vi "Reacquire Image.vi"(6 "Console Log in":refnum<class "Console Log.lvclass">, 7 "Gantry in":refnum<class "Gantry Class.lvclass">, 8 "error in":errorcluster, 10 "Chuck":i32, 11 "Fiducial Image In":T2) -> (0 "error out":errorcluster, 3 "Fiducial Image Out":T2, 4 "Console Log out":refnum<class "Console Log.lvclass">, 5 "Gantry out":refnum<class "Gantry Class.lvclass">)   [LabVIEW 2011]
uses:
  Shared Components/Utils/Type Definitions/Fiducial Image.ctl
  Shared Components/Vec3d Class/Vec3d Class.lvclass
  Shared Components/Utils/Type Definitions/Physical Image.ctl
  <vilib>/vision/Image Controls.llb/IMAQ Image.ctl
  Shared Components/Utils/Type Definitions/Fiducial with Source.ctl
  Shared Components/Gantry Class/Gantry Class.lvclass
  UI Classes/Console Log/Console Log.lvclass
  Shared Components/Config Manager Class/Type Definitions/Camera Enum.ctl
panel:
  out "Current Position":cluster{"X":dbl, "Y":dbl, "Z":dbl}
  in  "Accept":bool
  out "Preview":T1(plugin-control)
  # "Use MPG To locate fiducial\nand bring it into focus.\n\nClick \"Accept\" when\nsatisfied."
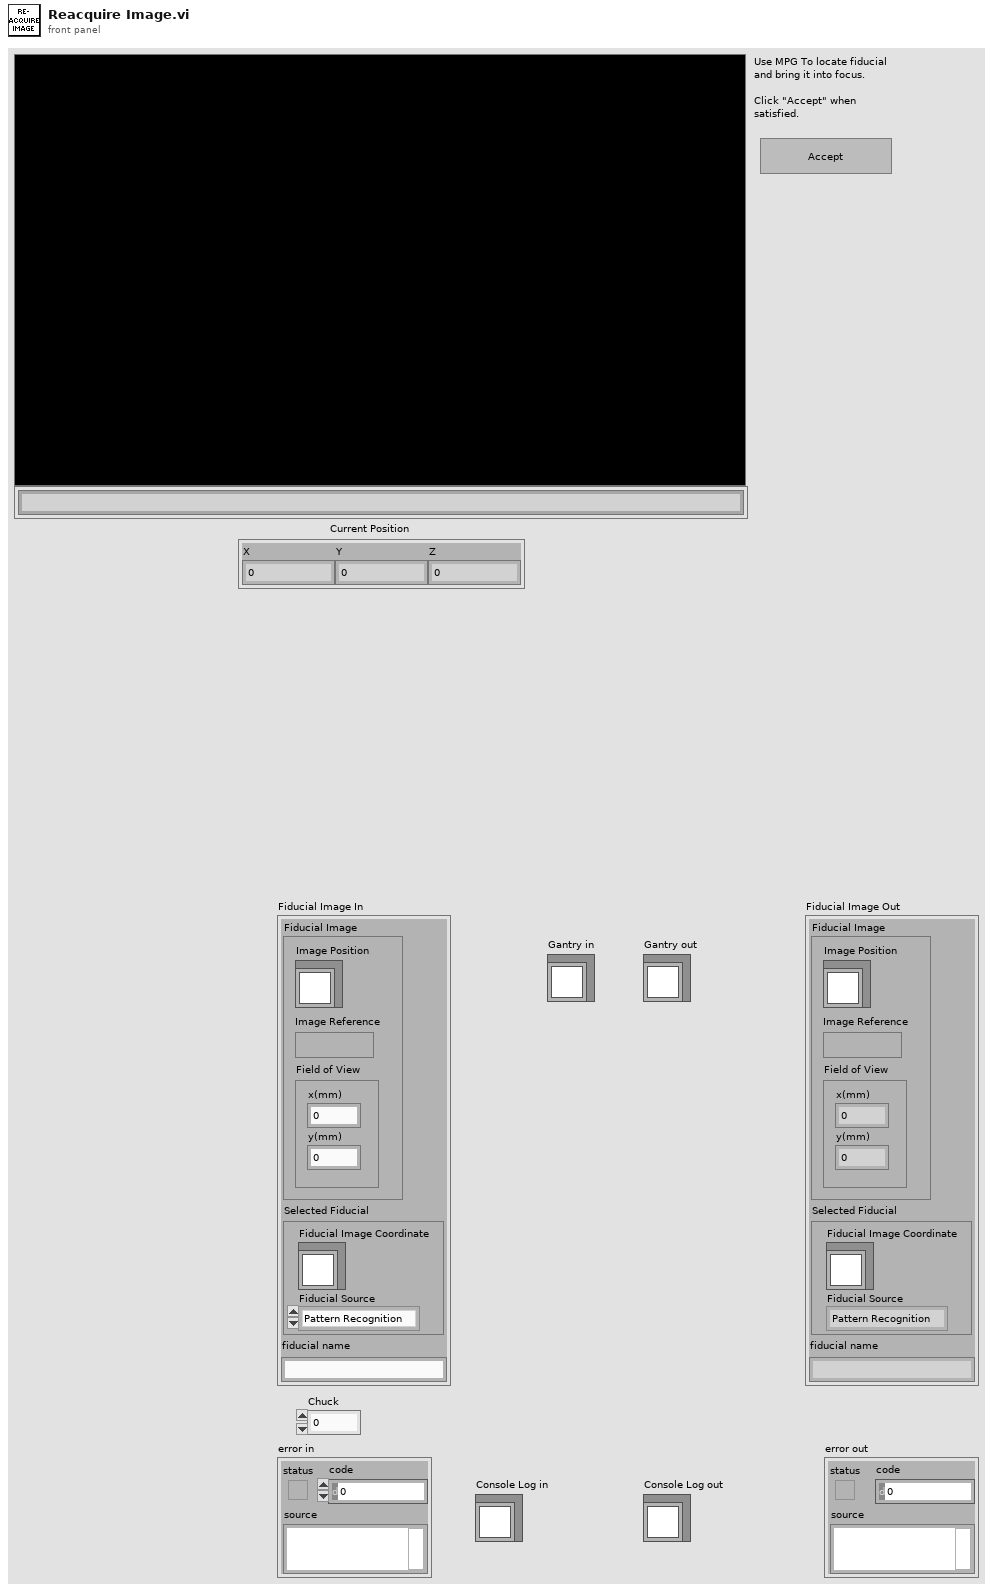
[diagram p1: front panel]
types:
  T1 = typedef "IMAQ Image.ctl" = refnum<image>
  T2 = typedef "Fiducial Image.ctl" = cluster{"Fiducial Image":T3, "Selected Fiducial":T4, "fiducial name":string}
  T3 = typedef "Physical Image.ctl" = cluster{"Image Position":refnum<class "Vec3d Class.lvclass">, "Image Reference":T1, "Field of View":cluster{"x(mm)":dbl, "y(mm)":dbl}}
  T4 = typedef "Fiducial with Source.ctl" = cluster{"Fiducial Image Coordinate":refnum<class "Vec3d Class.lvclass">, "Fiducial Source":enum16{"Pattern Recognition", "User", "Error", "Default"}}
  T5 = enum16{"Pattern Recognition", "User", "Error", "Default"}
  T6 = typedef "Camera Enum.ctl" = enum16{"GANTRY HEAD", "NEEDLE CALIBRATION X", "NEEDLE CALIBRATION Y"}
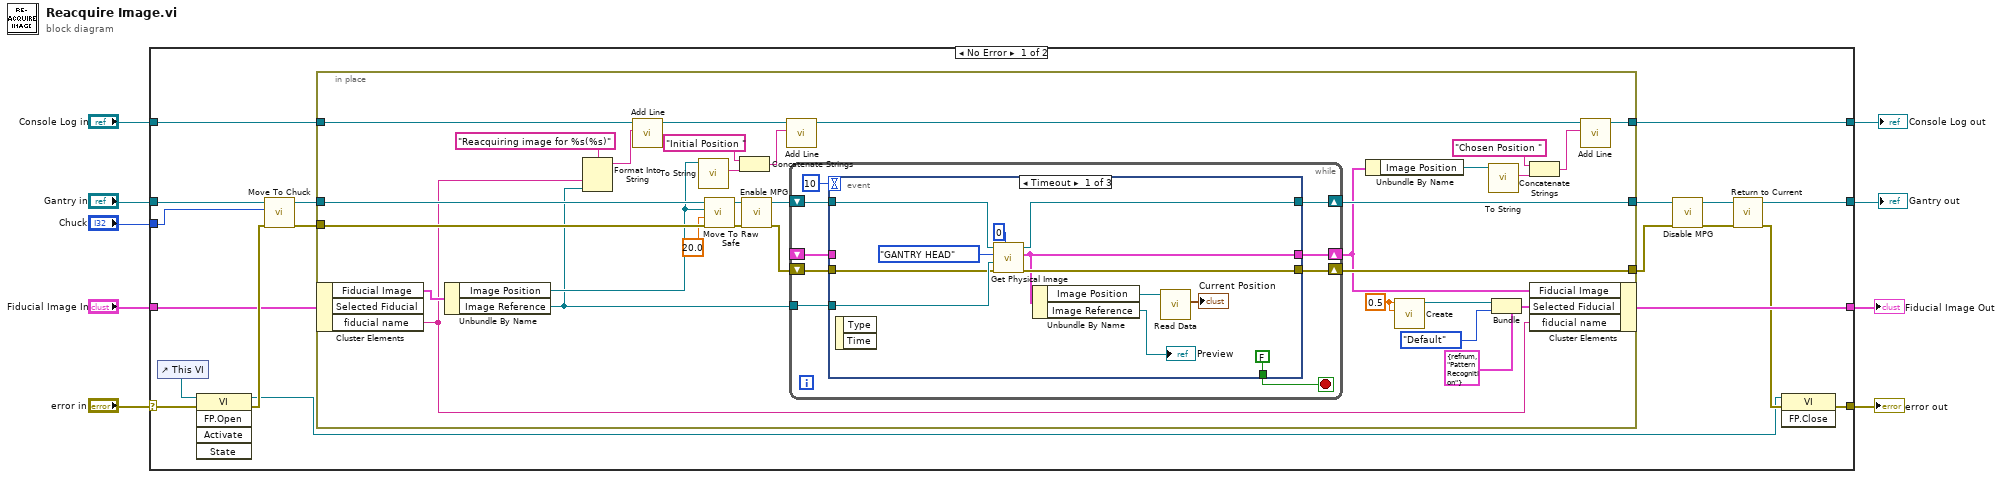
[diagram p0: block diagram]
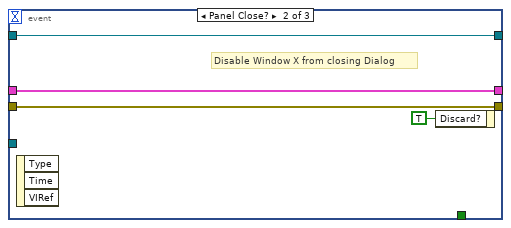
[diagram p2: hidden frame]
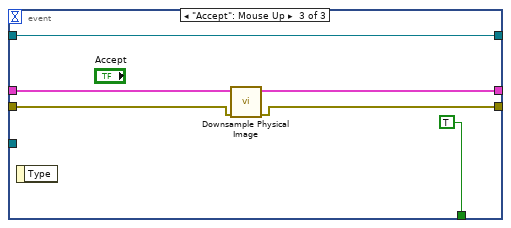
[diagram p3: hidden frame]
diagram:
  n1 = case shown="No Error" "error in" {
    selector: "error in" -> [w27 w95]
    tunnel: [w13 w95] -> w8
    tunnel: "Fiducial Image In" -> [w22 w93]
    tunnel: "Gantry in" -> [w26 w94]
    tunnel: [w16 w94] -> w5
    tunnel: "Chuck" -> [w24 _]
    tunnel: [w20 w93] -> w3
    tunnel: "Console Log in" -> [w11 w92]
    tunnel: [w10 w92] -> w1
    frame No Error {
      n2 = control-ref of="This VI"() -> (w28:refnum<vi>)
      n3 = invoke class="VI" method="FP.Open"(reference=w28, error in=w27) -> (reference out=w12:refnum<vi>, error out=w25:errorcluster)  [unwired: 3 in, 3 out]
      n4 = call-dynamic "Move To Chuck.vi"("error in"=w25, "Chuck"=w24, "Gantry in"=w26) -> ("error out"=w21:errorcluster, "Gantry out"=w23:refnum<class "Gantry Class.lvclass">)  [unwired: 7 in]
      n5 = in-place {
        in-place-border: w23 -> [w60]
        in-place-border: w21 -> [w59]
        in-place-border: [w53] -> w19
        in-place-border: [w52] -> w18
        in-place-border: w11 -> [w46]
        in-place-border: [w35] -> w10
        w49 = 0.5 ("X")
        n6 = in-place-cluster #1(w22) -> ("Fiducial Image"=w54:T3, "fiducial name"=w31:string)  [unwired: 1 out]
        n7 = Unbundle By Name(w54) -> ("Image Position"=w45:refnum<class "Vec3d Class.lvclass">, "Image Reference"=w30:T1)
        n8 = Format Into String(format string="Reacquiring image for %s(%s)", w31, w30) -> (resulting string=w32:string)  [unwired: 2 in, 1 out]
        n9 = call "Add Line.vi"("String"=w32, "Console Log in"=w46) -> ("Console Log out"=w44:refnum<class "Console Log.lvclass">)  [unwired: 8 in, 1 out]
        n10 = call "To String.vi"("Vec3d in"=w45) -> ("Vec3d String"=w43:string)  [unwired: 8 in, 2 out]
        n11 = call-dynamic "Move To Raw Safe.vi"("error in"=w59, "Speed(mm/s)"=20.0, "Destination"=w45, "Gantry in"=w60) -> ("error out"=w56:errorcluster, "Gantry out"=w58:refnum<class "Gantry Class.lvclass">)  [unwired: 6 in]
        n12 = Concatenate Strings("Initial Position ", w43) -> (w41:string)
        n13 = call-dynamic "Enable MPG.vi"("error in"=w56, "Gantry in"=w58) -> ("error out"=w55:errorcluster, "Gantry out"=w57:refnum<class "Gantry Class.lvclass">)  [unwired: 8 in]
        n14 = call "Add Line.vi"("String"=w41, "Console Log in"=w44) -> ("Console Log out"=w36:refnum<class "Console Log.lvclass">)  [unwired: 8 in, 1 out]
        n15 = while {
          tunnel: w30 -> [w66]
          shift-right: [w63] -> w53
          shift-left: w57 -> [w67]
          shift-right: [w62] -> w38
          shift-left: _ -> [w61]
          shift-right: [w64] -> w52
          shift-left: w55 -> [w65]
          stop <- w68 stop-if-true
          n16 = event shown="[0] Timeout" {
            selector: _ -> [_ _ _]
            dyn-events: _ -> [_ _ _]
            timeout: 10 -> [_ _ _]
            tunnel: [FALSE _ TRUE] -> w68
            tunnel: w67 -> [w80 w84 w90]
            tunnel: w66 -> [w77 _ _]
            tunnel: w65 -> [w76 w82 w87]
            tunnel: [w72 w82 w86] -> w64
            tunnel: [w71 w84 w90] -> w63
            tunnel: [w70 w83 w88] -> w62
            tunnel: w61 -> [_ w83 w89]
            event Timeout {
              n17 = event-data() -> ()  [unwired: 1 in, 2 out]
              n18 = call-dynamic "Get Physical Image.vi"("Delay(milliseconds)"=0, "error in"=w76, "Image In"=w77, "Camera Name"=Camera_Enum."GANTRY HEAD", "Gantry in"=w80) -> ("error out"=w72:errorcluster, "Physical Image"=w70:T3, "Gantry out"=w71:refnum<class "Gantry Class.lvclass">)  [unwired: 4 in]
              n19 = Unbundle By Name(w70) -> ("Image Position"=w74:refnum<class "Vec3d Class.lvclass">, "Image Reference"=→"Preview":T1)
              n20 = call-dynamic "Read Data.vi"("Vec3d Class in"=w74) -> ("Data"=→"Current Position":cluster{"X":dbl, "Y":dbl, "Z":dbl})  [unwired: 8 in, 2 out]
            }
            event Panel Close? {
              # "Disable Window X from closing Dialog"
              n21 = event-data() -> ()  [unwired: 1 in, 3 out]
              n22 = event-data("Discard?"=TRUE) -> ()  [unwired: 1 in, 1 out]
            }
            event "Accept": Mouse Up {
              n23 = event-data() -> ()  [unwired: 1 in, 1 out]
              n24 = call "Downsample Physical Image.vi"("error in"=w87, "Physical Image In"=w89) -> ("error out"=w86:errorcluster, "Physical Image Out"=w88:T3)  [unwired: 8 in]
            }
          }
        }
        n25 = Unbundle By Name(w38) -> ("Image Position"=w37:refnum<class "Vec3d Class.lvclass">)
        n26 = call "Create.vi"("Y"=w49, "X"=w49) -> ("Vec3d Class out"=w50:refnum<class "Vec3d Class.lvclass">)  [unwired: 8 in, 1 out]
        n27 = call "To String.vi"("Vec3d in"=w37) -> ("Vec3d String"=w40:string)  [unwired: 8 in, 2 out]
        n28 = Bundle(cluster=T4 {"Fiducial Image Coordinate"=refnum, "Fiducial Source"=enum."Pattern Recognition"} ("Selected Fiducial"), "Fiducial Image Coordinate"=w50, "Fiducial Source"=T5."Default") -> (w47:T4)
        n29 = Concatenate Strings("Chosen Position ", w40) -> (w34:string)
        n30 = in-place-cluster #1("Fiducial Image"=w38, "Selected Fiducial"=w47, "fiducial name"=w31) -> (w20:T2)
        n31 = call "Add Line.vi"("String"=w34, "Console Log in"=w36) -> ("Console Log out"=w35:refnum<class "Console Log.lvclass">)  [unwired: 8 in, 1 out]
      }
      n32 = call-dynamic "Disable MPG.vi"("error in"=w18, "Gantry in"=w19) -> ("error out"=w15:errorcluster, "Gantry out"=w17:refnum<class "Gantry Class.lvclass">)  [unwired: 8 in]
      n33 = call-dynamic "Return to Current.vi"("error in"=w15, "Gantry in"=w17) -> ("error out"=w14:errorcluster, "Gantry out"=w16:refnum<class "Gantry Class.lvclass">)  [unwired: 8 in]
      n34 = invoke class="VI" method="FP.Close"(reference=w12, error in=w14) -> (error out=w13:errorcluster)  [unwired: 1 in, 2 out]
    }
    frame Error {
    }
  }
  "Fiducial Image Out" <- w3
  "error out" <- w8
  "Gantry out" <- w5
  "Console Log out" <- w1
